vi "Active channels.vi"() -> ()   [LabVIEW 2017]
panel:
  out "Actual sampling time":dbl
  out "Ch2 Active":bool
  out "Ch1 Active":bool
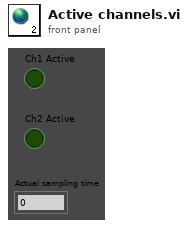
[diagram p1: front panel]
diagram:
